vi "GetType.vi"(8 "error in (no error)":errorcluster, 11 "Get Auto Range Value [ARV] Msg":refnum<class "Get Auto Range Value [ARV] Msg.lvclass">) -> (0 "error out":errorcluster, 2 "Data Sample":variant, 3 "Get Auto Range Value [ARV] Msg":refnum<class "Get Auto Range Value [ARV] Msg.lvclass">)   [LabVIEW 2015, in "CS++DMM.lvlib" / "Get Auto Range Value [ARV] Msg.lvclass"]
uses:
  Get Auto Range Value [ARV] Msg.lvclass
  Get Auto Range Value [ARV] Msg.lvclass/Get Auto Range Value [ARV] Msg.ctl
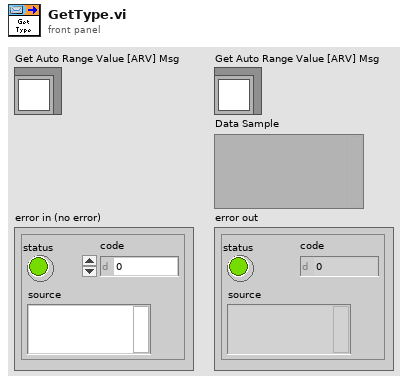
[diagram p1: front panel]
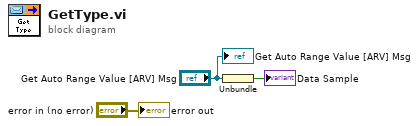
[diagram p0: block diagram]
diagram:
  n1 = Unbundle("Get Auto Range Value [ARV] Msg") -> (→"Data Sample":bool)
  "error out" <- "error in (no error)"
  "Get Auto Range Value [ARV] Msg" <- "Get Auto Range Value [ARV] Msg"
